vi "Parse Serial Data.vi"(8 "error in":errorcluster, 11 "Buffer in":string) -> (0 "error out":errorcluster, 2 "cluster":T1, 3 "Buffer out":string)   [LabVIEW 2019, in "PGC2D.lvlib"]
uses:
  PGC2D.lvlib
  sandbox/Instrument.AML.GetAll--Cluster.ctl
  <vilib>/Utility/error.llb/Error Cluster From Error Code.vi
  <vilib>/ErrorRing/Error Ring.xnode
panel:
  out "valid start characters?":bool
  out "valid end characters?":bool
  out "valid checksum?":bool
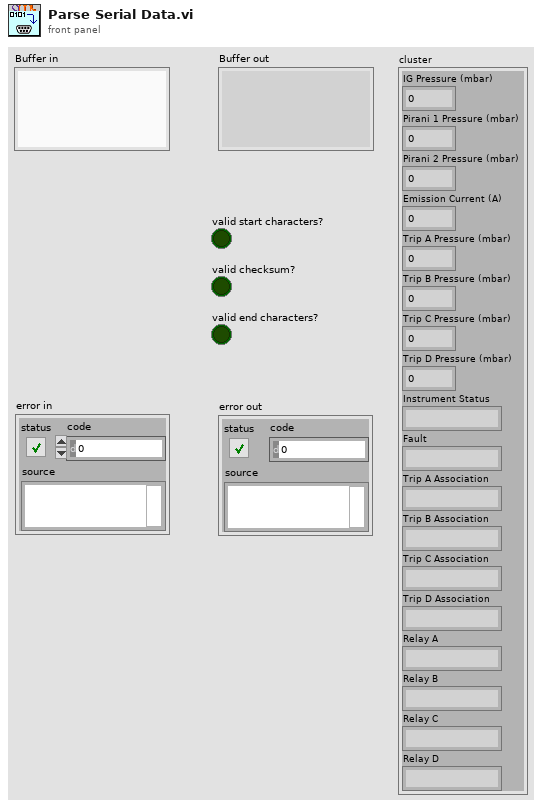
[diagram p1: front panel]
types:
  T1 = typedef "Instrument.AML.GetAll--Cluster.ctl" = cluster{"IG Pressure (mbar)":dbl, "Pirani 1 Pressure (mbar)":dbl, "Pirani 2 Pressure (mbar)":dbl, "Emission Current (A)":dbl, "Trip A Pressure (mbar)":dbl, "Trip B Pressure (mbar)":dbl, "Trip C Pressure (mbar)":dbl, "Trip D Pressure (mbar)":dbl, "Instrument Status":string, "Fault":string, "Trip A Association":string, "Trip B Association":string, "Trip C Association":string, "Trip D Association":string, "Relay A":string, "Relay B":string, "Relay C":string, "Relay D":string}
  T2 = enum16{"Relay A", "Relay B", "Relay C", "Relay D"}
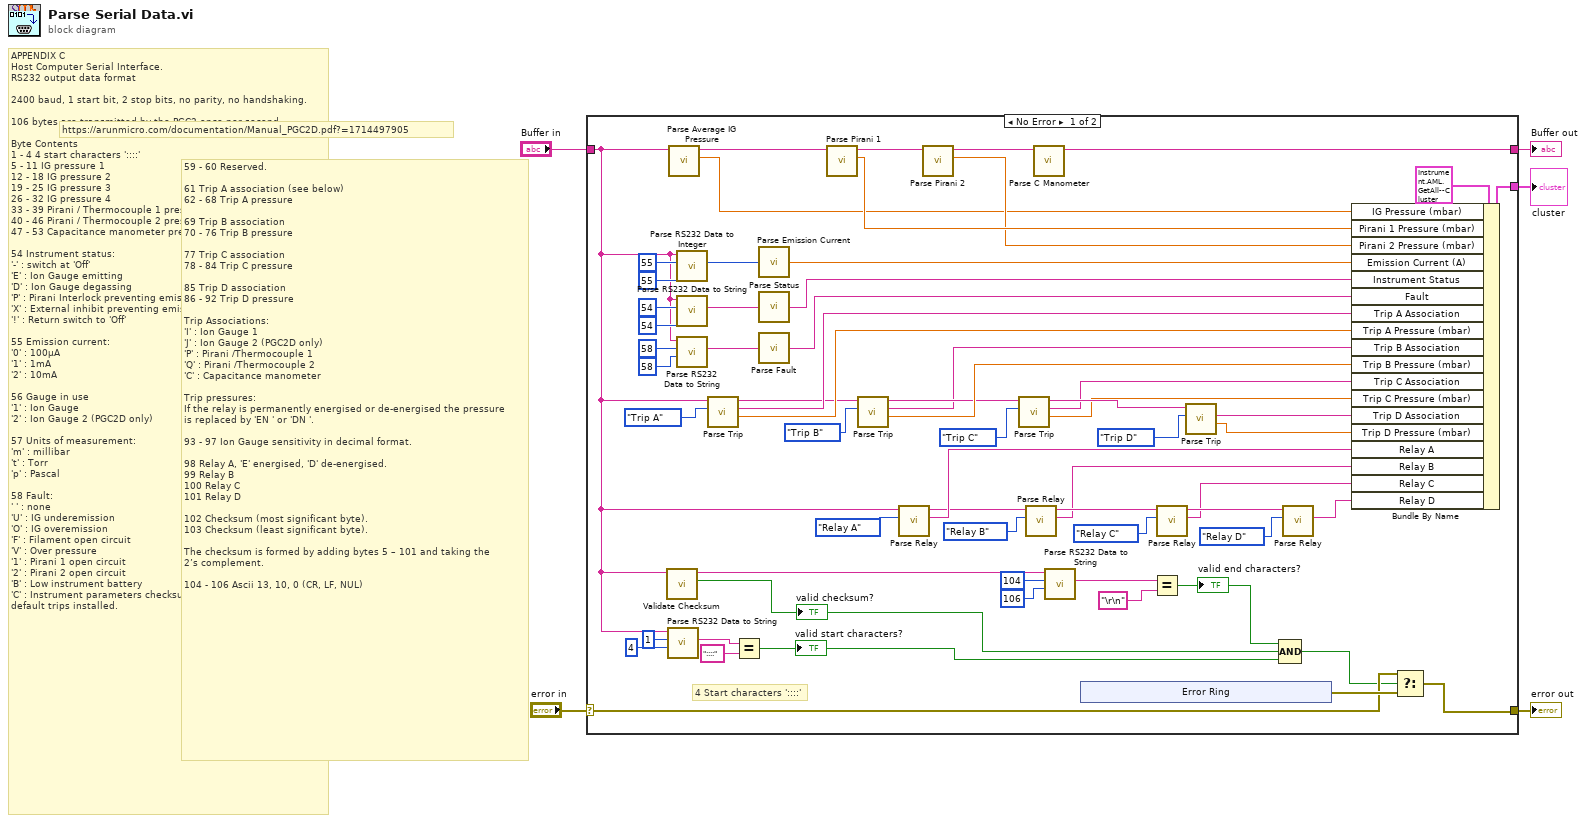
[diagram p0: block diagram]
diagram:
  # "https://arunmicro.com/documentation/Manual_PGC2D.pdf?=1714497905"
  # "59 - 60 Reserved.\n\n61 Trip A association (see below)\n62 - 68 Trip A pressure\n\n69 Trip B association\n70 - 76 Trip B pressure\n\n77 Trip C association\n78 - 84 Trip C pressure\n\n85 Trip D association\n86 - 92 Trip D pressure\n\nTrip Associations:\n'I' : Ion Gauge 1\n'J' : Ion Gauge 2 (PGC2D only)\n'P' : Pirani /Thermocouple 1\n'Q' : Pirani /Thermocouple 2\n'C' : Capacitance manometer\n\nTrip pressures:\nIf the relay is permanently energised or de-energised the pressure\nis replaced by 'EN ' or 'DN '.\n\n93 - 97 Ion Gauge sensitivity in decimal format.\n\n98 Relay A, 'E' energised, 'D' de-energised.\n99 Relay B\n100 Relay C\n101 Relay D\n\n102 Checksum (most significant byte).\n103 Checksum (least significant byte).\n\nThe checksum is formed by adding bytes 5 – 101 and taking the\n2’s complement.\n\n104 - 106 Ascii 13, 10, 0 (CR, LF, NUL)"
  # "APPENDIX C\nHost Computer Serial Interface.\nRS232 output data format\n\n2400 baud, 1 start bit, 2 stop bits, no parity, no handshaking.\n\n106 bytes are transmitted by the PGC2 once per second.\n\nByte Contents\n1 - 4 4 start characters '::::'\n5 - 11 IG pressure 1\n12 - 18 IG pressure 2\n19 - 25 IG pressure 3\n26 - 32 IG pressure 4\n33 - 39 Pirani / Thermocouple 1 pressure\n40 - 46 Pirani / Thermocouple 2 pressure\n47 - 53 Capacitance manometer pressure\n\n54 Instrument status:\n'-' : switch at 'Off'\n'E' : Ion Gauge emitting\n'D' : Ion Gauge degassing\n'P' : Pirani Interlock preventing emission / degas\n'X' : External inhibit preventing emission / degas\n'!' : Return switch to 'Off'\n\n55 Emission current:\n'0' : 100µA\n'1' : 1mA\n'2' : 10mA\n\n56 Gauge in use\n'1' : Ion Gauge\n'2' : Ion Gauge 2 (PGC2D only)\n\n57 Units of measurement:\n'm' : millibar\n't' : Torr\n'p' : Pascal\n\n58 Fault:\n' ' : none\n'U' : IG underemission\n'O' : IG overemission\n'F' : Filament open circuit\n'V' : Over pressure\n'1' : Pirani 1 open circuit\n'2' : Pirani 2 open circuit\n'B' : Low instrument battery\n'C' : Instrument parameters checksum incorrect,\ndefault trips installed."
  n1 = case shown="No Error" "error in" {
    selector: "error in" -> [w49 w74]
    tunnel: "Buffer in" -> [w6 w73]
    tunnel: [w57 _] -> w4
    tunnel: [w48 w74] -> w2
    tunnel: [w9 w73] -> w1
    frame No Error {
      # "4 Start characters '::::'"
      n2 = call "Validate Checksum.vi"("bytes in"=w6) -> ("Boolean"=w41:bool, "bytes out"=w7:string)  [unwired: 9 in]
      "valid checksum?" <- w41
      n3 = call "Parse RS232 Data to String.vi"("AML end byte"=4 ("length (rest)"), "AML start byte"=1 ("offset (0)"), "bytes in"=w6) -> ("string data"=w43:string)  [unwired: 7 in, 1 out]
      n4 = call "Parse Average IG Pressure.vi"("Buffer in"=w6) -> ("mean"=w8:dbl, "Buffer out"=w10:string)  [unwired: 9 in]
      n5 = call "Parse RS232 Data to Integer.vi"("AML end byte"=55, "AML start byte"=55, "bytes in"=w6) -> ("I32 data"=w59:i32)  [unwired: 7 in, 1 out]
      n6 = call "Parse RS232 Data to String.vi"("AML end byte"=54, "AML start byte"=54, "bytes in"=w6) -> ("string data"=w64:string)  [unwired: 7 in, 1 out]
      n7 = call "Parse RS232 Data to String.vi"("AML end byte"=58, "AML start byte"=58, "bytes in"=w6) -> ("string data"=w36:string)  [unwired: 7 in, 1 out]
      n8 = call "Parse Trip.vi"("Trip"=enum16{"Trip A", "Trip B", "Trip C", "Trip D"}."Trip A", "Buffer in"=w6) -> ("Trip Pressure"=w34:dbl, "Trip Association"=w35:string, "Buffer out"=w33:string)  [unwired: 7 in]
      n9 = Equal?(x=w43, y="::::" ("substring")) -> (x = y?=w40:bool)
      "valid start characters?" <- w40
      n10 = call "Parse Emission Current.vi"("Numeric"=w59) -> ("current (A)"=w55:dbl)
      n11 = call "Parse Status.vi"("Buffer in"=w64) -> ("status"=w37:string)
      n12 = call "Parse Fault.vi"("Buffer in"=w36) -> ()  [unwired: 1 out]
      n13 = call "Parse Pirani 1.vi"("Buffer in"=w10) -> ("DBL data"=w65:dbl, "bytes out"=w67:string)  [unwired: 9 in]
      n14 = call "Parse Trip.vi"("Trip"=enum16{"Trip A", "Trip B", "Trip C", "Trip D"}."Trip B", "Buffer in"=w33) -> ("Trip Pressure"=w31:dbl, "Trip Association"=w22:string, "Buffer out"=w29:string)  [unwired: 7 in]
      n15 = call "Parse Relay.vi"("Relay"=T2."Relay A", "Buffer in"=w6) -> ("relay"=w20:string, "Buffer out"=w19:string)  [unwired: 8 in]
      n16 = call "Parse Pirani 2.vi"("bytes in"=w67) -> ("DBL data"=w56:dbl, "bytes out"=w66:string)  [unwired: 9 in]
      n17 = call "Parse Trip.vi"("Trip"=enum16{"Trip A", "Trip B", "Trip C", "Trip D"}."Trip C", "Buffer in"=w29) -> ("Trip Pressure"=w25:dbl, "Trip Association"=w26:string, "Buffer out"=w27:string)  [unwired: 7 in]
      n18 = call "Parse Relay.vi"("Relay"=T2."Relay B", "Buffer in"=w19) -> ("relay"=w13:string, "Buffer out"=w18:string)  [unwired: 8 in]
      n19 = call "Parse C Manometer.vi"("bytes in"=w66) -> ("bytes out"=w9:string)  [unwired: 9 in, 1 out]
      n20 = call "Parse RS232 Data to String.vi"("AML end byte"=106, "AML start byte"=104, "bytes in"=w7) -> ("string data"=w51:string)  [unwired: 7 in, 1 out]
      n21 = xnode "Error Ring"() -> ("error out"=w50:errorcluster)
      n22 = Equal?(x=w51, y="\r\n" ("string data")) -> (x = y?=w42:bool)
      "valid end characters?" <- w42
      n23 = call "Parse Relay.vi"("Relay"=T2."Relay C", "Buffer in"=w18) -> ("relay"=w12:string, "Buffer out"=w17:string)  [unwired: 8 in]
      n24 = call "Parse Trip.vi"("Trip"=enum16{"Trip A", "Trip B", "Trip C", "Trip D"}."Trip D", "Buffer in"=w27) -> ("Trip Pressure"=w21:dbl, "Trip Association"=w24:string)  [unwired: 7 in, 1 out]
      n25 = Compound Arithmetic op=AND(w42, w41, w40) -> (w39:bool)
      n26 = call "Parse Relay.vi"("Relay"=T2."Relay D", "Buffer in"=w17) -> ("relay"=w11:string)  [unwired: 8 in, 1 out]
      n27 = Bundle By Name(cluster=T1 {"IG Pressure (mbar)"=0.0, "Pirani 1 Pressure (mbar)"=0.0, "Pirani 2 Pressure (mbar)"=0.0, "Emission Current (A)"=0.0, "Trip A Pressure (mbar)"=0.0, "Trip B Pressure (mbar)"=0.0, "Trip C Pressure (mbar)"=0.0, "Trip D Pressure (mbar)"=0.0, "Instrument Status"="", "Fault"="", "Trip A Association"="", "Trip B Association"="", "Trip C Association"="", "Trip D Association"="", "Relay A"="", "Relay B"="", "Relay C"="", "Relay D"=""}, "IG Pressure (mbar)"=w8, "Pirani 1 Pressure (mbar)"=w65, "Pirani 2 Pressure (mbar)"=w56, "Emission Current (A)"=w55, "Instrument Status"=w37, "Fault"=w36, "Trip A Association"=w35, "Trip A Pressure (mbar)"=w34, "Trip B Association"=w22, "Trip B Pressure (mbar)"=w31, "Trip C Association"=w26, "Trip C Pressure (mbar)"=w25, "Trip D Association"=w24, "Trip D Pressure (mbar)"=w21, "Relay A"=w20, "Relay B"=w13, "Relay C"=w12, "Relay D"=w11) -> (w57:T1)
      n28 = Select(t=w49, s=w39, f=w50) -> (s? t:f=w48:errorcluster)
    }
    frame Error {
    }
  }
  "cluster" <- w4
  "error out" <- w2
  "Buffer out" <- w1
